vi "Simple UDP - Sender.vi"() -> ()   [LabVIEW 2017]
doc: "The UDP protocol differs from TCP in that there is no error-checking with the packets of information that are sent, and thus no guarantee whatsoever that an intended recipient will actually receive a given piece of data.\n\nUDP does offer the ability to \"broadcast\" data across a network--simply specify an IP Address of all ones (255.255.255.255) to attempt to broadcast information network-wide. Keep in mind that routers and other network hardware will generally refuse to forward the broadcast beyond certain points, so the extent of the broadcast will in practice be limited."
panel:
  out "문자열":string
  in  "Stop":bool
  # "Overview: Demonstrates the use of the UDP functions to send data over a UDP connection.\nInstructions:\n1. Run the VI.\n2. Open Simple UDP - Receiver.vi and follow the instructions on its front panel.\n3. Click Stop to stop the VI."
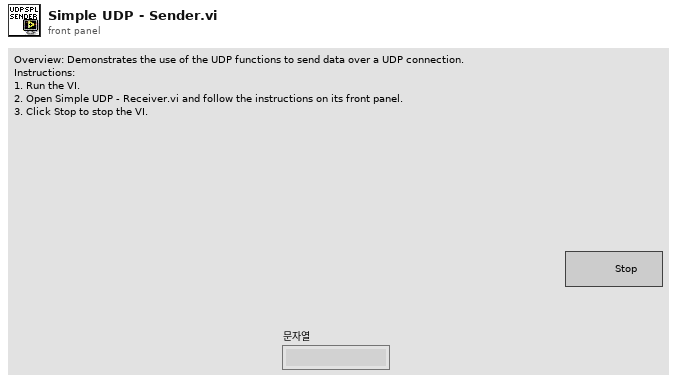
[diagram p1: front panel]
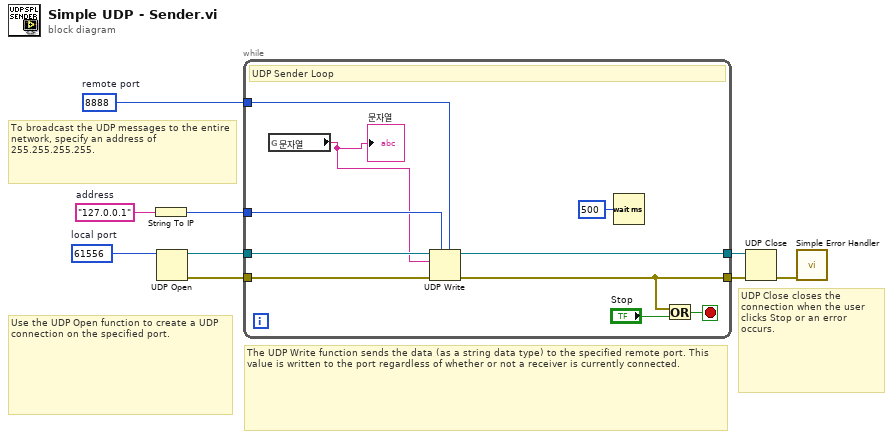
[diagram p0: block diagram]
diagram:
  w1 = u16 8888  # remote port
  w2 = u16 61556  # local port
  w7 = "127.0.0.1"  # address
  # "To broadcast the UDP messages to the entire network, specify an address of 255.255.255.255."
  # "UDP Close closes the connection when the user clicks Stop or an error occurs."
  # "The UDP Write function sends the data (as a string data type) to the specified remote port. This value is written to the port regardless of whether or not a receiver is currently connected."
  # "Use the UDP Open function to create a UDP connection on the specified port."
  n1 = String To IP(1:w7) -> (0:w5:u32)
  n2 = UDP Open(11:w2) -> (port=w4:refnum<k16>, 0:w3:errorcluster)  [unwired: 4 in, 1 out]
  n3 = while {
    tunnel: [w14] -> w8
    tunnel: w4 -> [w19]
    tunnel: w3 -> [w18]
    tunnel: [w15] -> w9
    tunnel: w5 -> [w13]
    tunnel: w1 -> [w11]
    stop <- w17 stop-if-true
    # "UDP Sender Loop"
    n4 = global read "글로벌 1.vi" "문자열"() -> (w10:string)
    "문자열" <- w10
    n5 = UDP Write(address=w13, port or service name=w11, connection ID=w19, data in=w10, 8:w18) -> (error out=w14:errorcluster, 3:w15:refnum<k16>)  [unwired: 1 in]
    n6 = Wait (ms)(milliseconds to wait=u32 500) -> ()  [unwired: 1 out]
    n7 = Or(x=w14, y="Stop") -> (x .or. y?=w17:bool)
  }
  n8 = UDP Close(connection ID=w9, 8:w8) -> (error out=w6:errorcluster)  [unwired: 1 out]
  n9 = call <vilib>:"Simple Error Handler.vi"("error in (no error)"=w6) -> ()  [unwired: 4 in, 5 out]
